vi "Read pcap class.vi"(8 "error in (no error)":errorcluster, 11 "CAN_RW_CORE in":refnum<class "L2ENET_RW_CORE.lvclass">) -> (0 "error out":errorcluster, 2 "pcap class":refnum<class "pcap_Parse_Build_CIF.lvclass">, 3 "CAN_RW_CORE out":refnum<class "L2ENET_RW_CORE.lvclass">)   [LabVIEW 2021, in "L2ENET_RW_CORE.lvclass"]
uses:
  L2ENET_RW_CORE.lvclass
  L2ENET_RW_CORE.lvclass/L2ENET_RW_CORE.ctl
  <vilib>/CIF Foundation/CIF PCAP Parse and Build/pcap_Parse_Build_CIF.lvclass
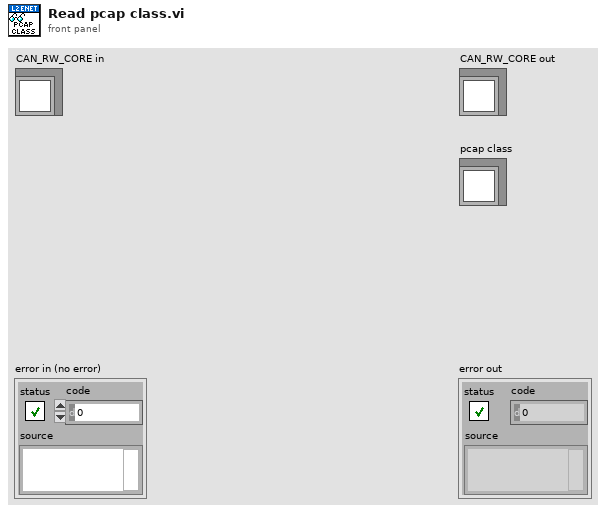
[diagram p1: front panel]
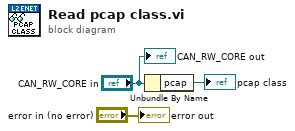
[diagram p0: block diagram]
diagram:
  n1 = Unbundle By Name("CAN_RW_CORE in") -> ("pcap"=→"pcap class":refnum<class "pcap_Parse_Build_CIF.lvclass">)
  "error out" <- "error in (no error)"
  "CAN_RW_CORE out" <- "CAN_RW_CORE in"
